vi "DI redefine.vi"(6 "conninfo":T4={"host"="localhost", "port"="5432", "client_encoding"="WIN1251", "dbname"="data", "user"="postgres", "password"=""}, 7 "KFM":string[](array[string]), 8 "error in (no error)":errorcluster, 9 "DIParamTable":string="fd_3", 10 "DIParameters":string[](array[string]), 11 "DI in":T1) -> (0 "error":errorcluster, 3 "DI out":T1)   [LabVIEW 2019, in "Inputs.lvlib"]
uses:
  Inputs.lvlib
  Ctl/DI.ctl
  Ctl/DI short.ctl
  Ctl/Parameter State.ctl
  Database/ctl/Coninfo.ctl
  Ctl/DIParamColumns.ctl
  Database/PostgreSQL2LabVIEW/libpqUtility/src/PQconnect.vi
  Database/PostgreSQL2LabVIEW/libpqUtility/src/PQclose.vi
  Database/select_initial_all.vi
  Database/PostgreSQL2LabVIEW/libpqlv/src/PQfinish.vi
  Database/PostgreSQL2LabVIEW/libpqlv/src/PQconnectdb.vi
  Database/PostgreSQL2LabVIEW/libpqlv/src/PQerrorMessage.vi
  Database/PostgreSQL2LabVIEW/libpqlv/src/PQstatus.vi
  <vilib>/dlg_ctls.llb/Space Constant.vi
  Database/PostgreSQL2LabVIEW/libpqUtility/src/PQgetTable.vi
  Database/Progress.vi
  Database/PostgreSQL.lvlib
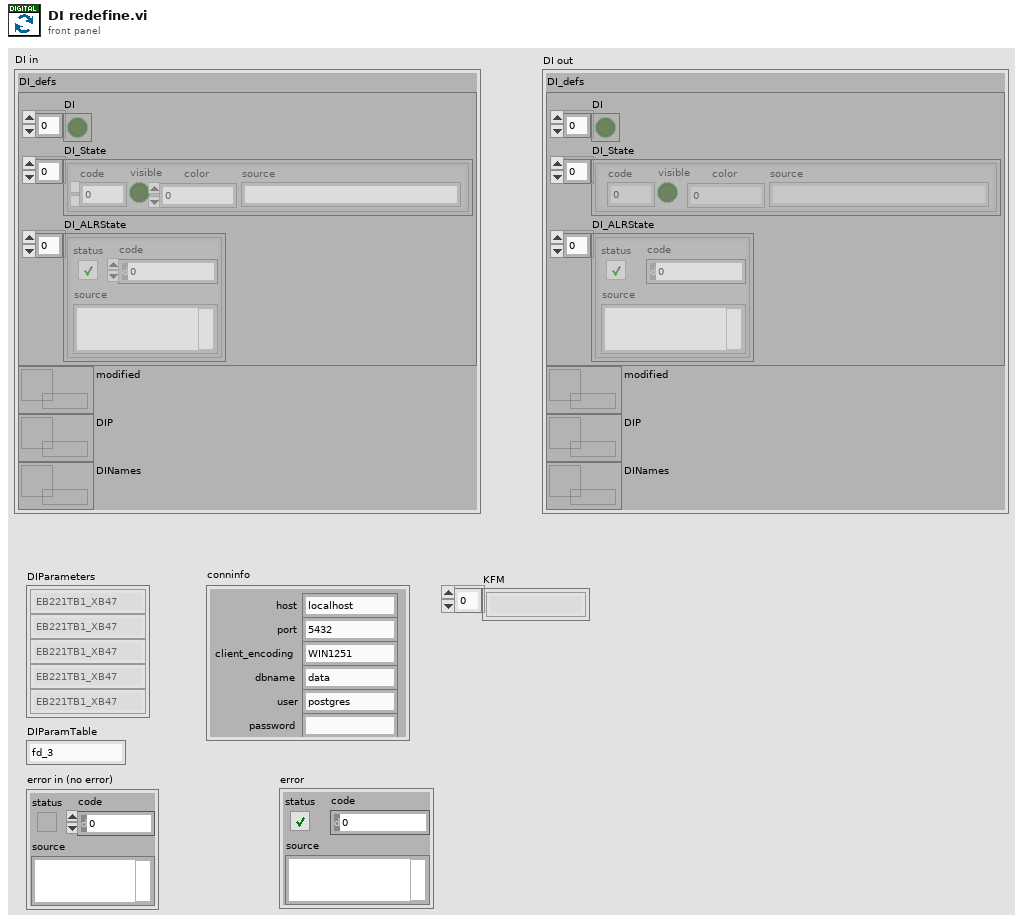
[diagram p1: front panel]
types:
  T1 = typedef "Inputs.lvlib/DI.ctl" = cluster{"DI_defs":T2, "modified":refnum<data-value>, "DIP":refnum<data-value>, "DINames":refnum<data-value>}
  T2 = typedef "Inputs.lvlib/DI short.ctl" = cluster{"DI":bool[], "DI_State":T3[], "DI_ALRState":errorcluster[]}
  T3 = typedef "Inputs.lvlib/Parameter State.ctl" = cluster{"code":i32, "visible":bool, "color":u32, "source":string}
  T4 = typedef "PostgreSQL.lvlib/Coninfo.ctl" = cluster{"host":string, "port":string, "client_encoding":string, "dbname":string, "user":string, "password":string}
  T5 = typedef "Inputs.lvlib/DIParamColumns.ctl" = enum16{"invert", "time_const", "module_fcode_full", "control_channel_num", "ip_adress", "fcode", "fcodef", "fcode_full", "fname"}
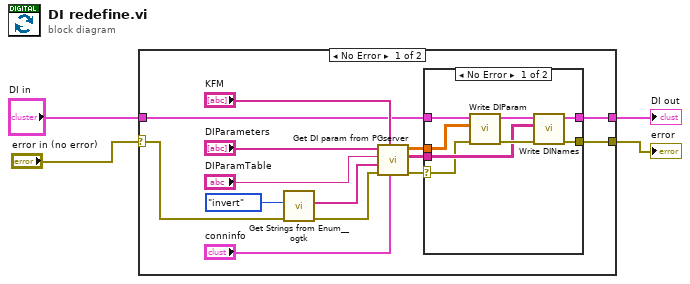
[diagram p0: block diagram]
diagram:
  n1 = case shown="No Error" "error in (no error)" {
    selector: "error in (no error)" -> [w12 w30]
    tunnel: [w5 w30] -> w4
    tunnel: "DI in" -> [w7 w29]
    tunnel: [w6 w29] -> w3
    frame No Error {
      n2 = call <userlib>:"Get Strings from Enum__ogtk.vi"("error in (no error)"=w12, "Enum"=DIParamColumns."invert" ("DIParamColumns")) -> ("error out"=w11:errorcluster, "Enum Strings"=w13:string[])  [unwired: 6 in, 2 out]
      n3 = call "Get DI param from PGserver.vi"("conninfo"="conninfo", "KFM"="KFM", "error in (no error)"=w11, "DIParamColumns"=w13, "DIParamTable"="DIParamTable", "DI_fcode_full"="DIParameters") -> ("error out"=w8:errorcluster, "Names table"=w9:string[][], "DIParameters table"=w10:dbl[][])  [unwired: 3 in]
      n4 = case shown="No Error" w8 {
        selector: w8 -> [w19 w27]
        tunnel: w10 -> [w20 _]
        tunnel: w9 -> [w21 _]
        tunnel: [w24 w27] -> w5
        tunnel: w7 -> [w26 w28]
        tunnel: [w25 w28] -> w6
        frame No Error {
          n5 = call "Write DIParam.vi"("error in (no error)"=w19, "DIParam"=w20, "DI in"=w26) -> ("error out"=w23:errorcluster, "DI out"=w22:T1)  [unwired: 7 in]
          n6 = call "Write DINames.vi"("error in (no error)"=w23, "DINames"=w21, "DI in"=w22) -> ("error out"=w24:errorcluster, "DI out"=w25:T1)  [unwired: 7 in]
        }
        frame Error {
        }
      }
    }
    frame Error {
    }
  }
  "DI out" <- w3
  "error" <- w4
